vi "Read PPMS T and B.vi"() -> (0 "Field":dbl=-0.001072365790605545, 1 "Temperature":dbl=138.3252)   [LabVIEW 2013]
doc: "This VI reads PPMS temperature and field remotely from the PPMS computer. Make sure IP address is correct before use."
panel:
  in  "IP Address":string="130.49.180.87"
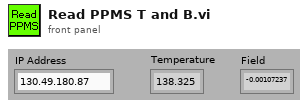
[diagram p1: front panel]
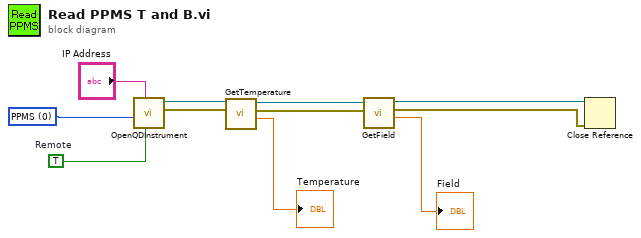
[diagram p0: block diagram]
diagram:
  w10 = TRUE  # Remote
  w9 = 0 items=["PPMS", "VersaLab", "DynaCool", "SVSM"] ("Instrument\nType")
  n1 = call <userlib>:"OpenQDInstrument.vi"("Remote"=w10, "IP Address"="IP Address", "Instrument Type"=w9) -> ("error out"=w7:errorcluster, "Instrument Ref"=w8:refnum<k24>)  [unwired: 5 in]
  n2 = call <userlib>:"GetTemperature.vi"("error in (no error)"=w7, "Instrument Ref In"=w8) -> ("Temperature"=→"Temperature":dbl, "error out"=w3:errorcluster, "Instrument Ref Out"=w5:refnum<k24>)  [unwired: 3 in, 2 out]
  n3 = call <userlib>:"GetField.vi"("error in (no error)"=w3, "Instrument Ref In"=w5) -> ("Field"=→"Field":dbl, "error out"=w2:errorcluster, "Instrument Ref Out"=w4:refnum<k24>)  [unwired: 3 in, 2 out]
  n4 = Close Reference(reference=w4, error in (no error)=w2) -> ()  [unwired: 1 out]
